vi "CMD_FINDFIDFOCUS.vi"(6 "Gantry in":refnum<class "Gantry.lvclass">, 8 "error in (no error)":errorcluster, 10 "Arguments":string[](array[string]), 11 "gScript Interpreter in":refnum<class "gScript Interpreter.lvclass">) -> (0 "error out":errorcluster, 3 "gScript Interpreter out":refnum<class "gScript Interpreter.lvclass">, 4 "Gantry out":refnum<class "Gantry.lvclass">)   [LabVIEW 2017, in "gScript Interpreter.lvclass"]
uses:
  gScript Interpreter.lvclass
  Shared Components/Vec3d Class/Vec3d.lvclass
  Shared Components/Gantry Class/Gantry.lvclass
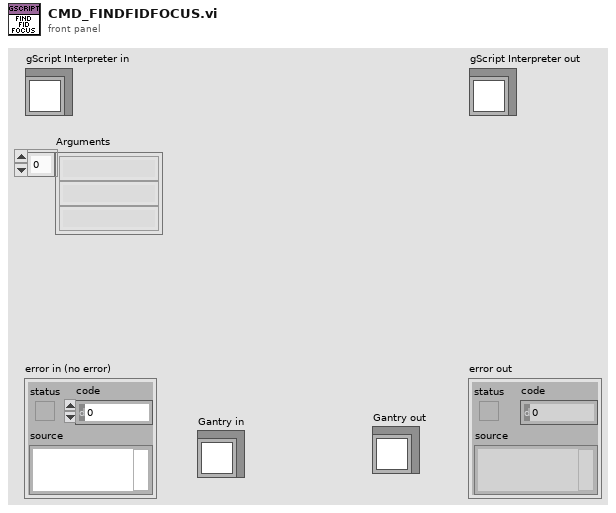
[diagram p1: front panel]
types:
  T1 = typedef "Physical Image.ctl" = cluster{"Image Position":refnum<class "Vec3d.lvclass">, "Image Reference":T2, "Field of View":cluster{"x(mm)":dbl, "y(mm)":dbl}}
  T2 = typedef "IMAQ Image.ctl" = refnum<image>
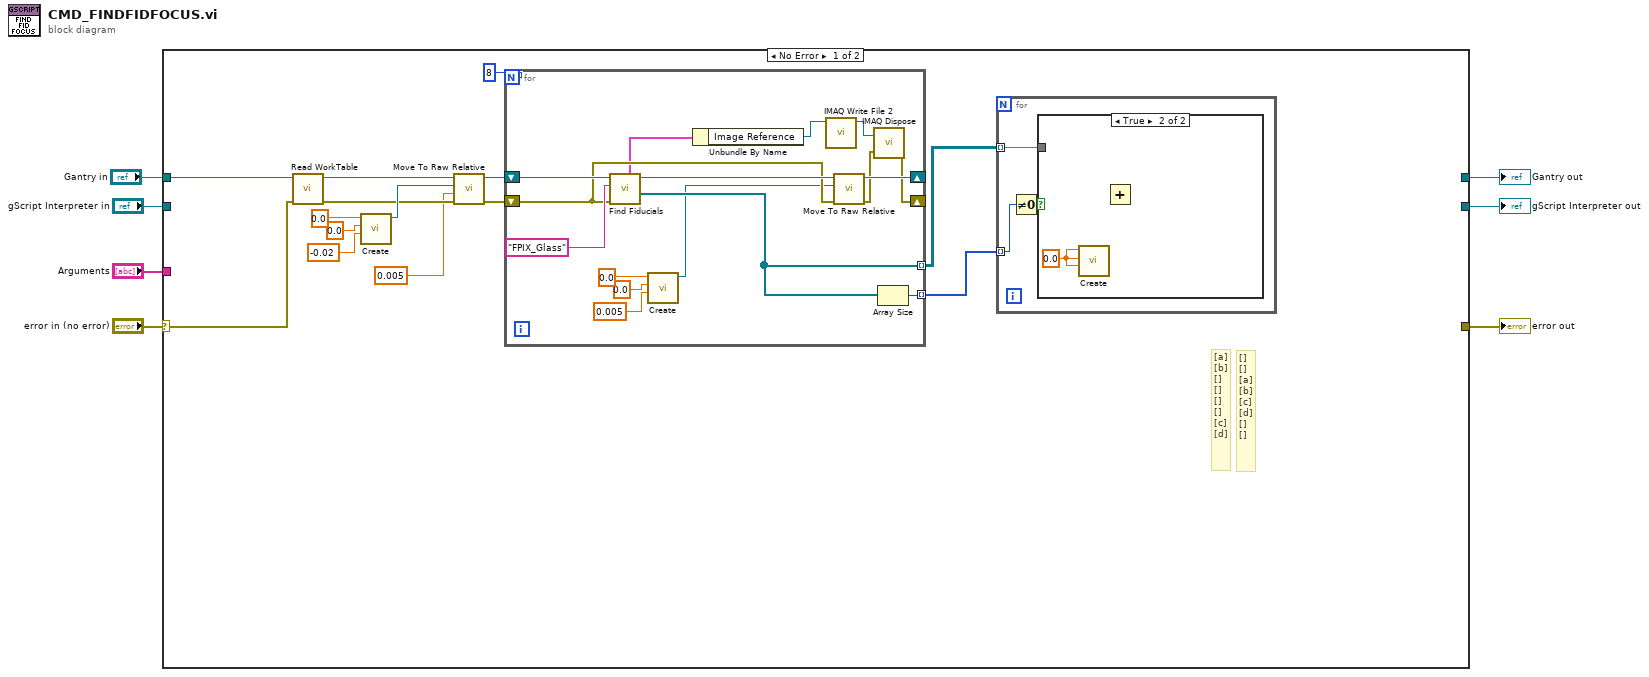
[diagram p0: block diagram]
diagram:
  n1 = case shown="No Error" "error in (no error)" {
    selector: "error in (no error)" -> [w20 w44]
    tunnel: [_ w44] -> w6
    tunnel: [_ w43] -> w4
    tunnel: "gScript Interpreter in" -> [_ w43]
    tunnel: "Arguments" -> [_ _]
    tunnel: "Gantry in" -> [w21 w42]
    tunnel: [_ w42] -> w1
    frame No Error {
      # "[]\n[]\n[a]\n[b]\n[c]\n[d]\n[]\n[]"
      # "[a]\n[b]\n[]\n[]\n[]\n[]\n[c]\n[d]"
      n2 = call-dynamic "Read WorkTable.vi"("error in"=w20, "Gantry Class in"=w21) -> ("error out"=w14:errorcluster, "Gantry Class out"=w19:refnum<class "Gantry.lvclass">)  [unwired: 7 in, 1 out]
      n3 = call "Create.vi"("Z"=-0.02, "Y"=0.0, "X"=0.0) -> ("Vec3d Class out"=w15:refnum<class "Vec3d.lvclass">)  [unwired: 7 in, 1 out]
      n4 = call-dynamic "Move To Raw Relative.vi"("error in"=w14, "Speed(mm/s)"=0.005, "Delta"=w15, "Gantry in"=w19) -> ("error out"=w10:errorcluster, "Gantry out"=w11:refnum<class "Gantry.lvclass">)  [unwired: 6 in]
      n5 = for {
        N: 8 -> [_]
        shift-right: [w36] -> _
        shift-left: w11 -> [w40]
        tunnel: [w39] -> w8 mode=indexing
        tunnel: [w38] -> w9 mode=indexing
        shift-right: [w32] -> _
        shift-left: w10 -> [w35]
        n6 = call "Find Fiducials.vi"("error in (no error)"=w35, "Fiducial Type"="FPIX_Glass", "Gantry in"=w40) -> ("Fiducial Physical Positions"=w39:refnum<class "Vec3d.lvclass">[], "Gantry out"=w37:refnum<class "Gantry.lvclass">, "Fiducial Image"=w34:T1)  [unwired: 4 in, 2 out]
        n7 = call "Create.vi"("Z"=0.005, "Y"=0.0, "X"=0.0) -> ("Vec3d Class out"=w28:refnum<class "Vec3d.lvclass">)  [unwired: 7 in, 1 out]
        n8 = Unbundle By Name(w34) -> ("Image Reference"=w26:T2)
        n9 = call-poly "IMAQ Write File 2"("Image"=w26) -> ("Image Out (duplicate)"=w27:T2)  [unwired: 9 in, 1 out]
        n10 = call-dynamic "Move To Raw Relative.vi"("error in"=w35, "Delta"=w28, "Gantry in"=w37) -> ("error out"=w33:errorcluster, "Gantry out"=w36:refnum<class "Gantry.lvclass">)  [unwired: 7 in]
        n11 = call "IMAQ Dispose"("Image"=w27, "error in (no error)"=w33) -> ("error out"=w32:errorcluster)  [unwired: 4 in]
        n12 = Array Size(array=w39) -> (size(s)=w38:i32)
      }
      n13 = for {
        tunnel: w9 -> [w23] mode=indexing
        tunnel: w8 -> [w22] mode=indexing
        n14 = Not Equal To 0?(x=w23) -> (x != 0?=w24:bool)
        n15 = case shown="True" w24 {
          tunnel: w22 -> [_ _]
          frame False {
          }
          frame True {
            w25 = 0.0
            n16 = call "Create.vi"("Z"=w25, "Y"=w25, "X"=w25) -> ()  [unwired: 7 in, 2 out]
            n17 = Add() -> ()  [unwired: 2 in, 1 out]
          }
        }
      }
    }
    frame Error {
    }
  }
  "error out" <- w6
  "gScript Interpreter out" <- w4
  "Gantry out" <- w1
